vi "libssh2_session_last_errno.vi"(8 "error in (no error)":errorcluster, 11 "session":T1) -> (0 "error out":errorcluster, 2 "error code":i32)   [LabVIEW 2013, in "libssh2.lvlib"]
doc: "Get the last error code for a session."
uses:
  libssh2.lvlib
  Session Refnum.ctl
  Global Settings.vi
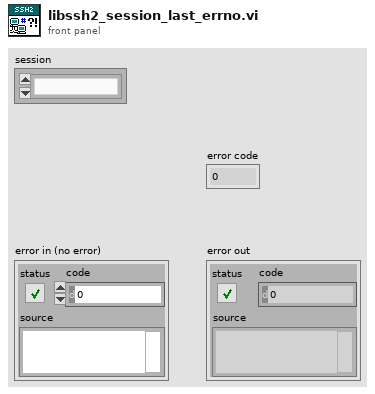
[diagram p1: front panel]
types:
  T1 = typedef "libssh2.lvlib/Session Refnum.ctl" = refnum<k1>
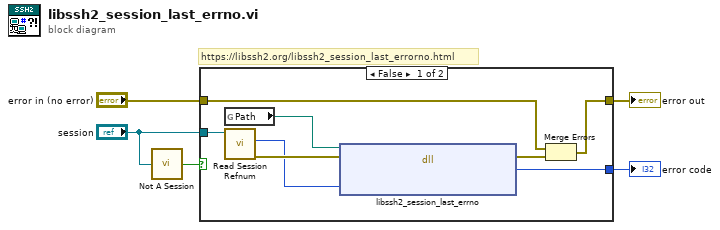
[diagram p0: block diagram]
diagram:
  # "https://libssh2.org/libssh2_session_last_errorno.html"
  n1 = call "Not A Session.vi"("session"="session") -> ("Not a Session?"=w1:bool)
  n2 = case shown="False" w1 {
    tunnel: [w8 w14] -> w5
    tunnel: [w13 _] -> w4
    tunnel: "error in (no error)" -> [w9 w14]
    tunnel: "session" -> [w11 _]
    frame False {
      n3 = global read "Global Settings.vi" "Path"() -> (w6:path)
      n4 = call "Read Session Refnum.vi"("session"=w11) -> ("error out"=w12:errorcluster, "LIBSSH2_SESSION*"=w10:u64)  [unwired: 6 in, 3 out]
      n5 = dll-call lib="?" fn="libssh2_session_last_errno"(path in=w6, error in=w12, "session"=w10) -> (error out=w7:errorcluster, "return value"=w13:i32)  [unwired: 2 in, 1 out]
      n6 = Merge Errors(w9, w7) -> (w8:errorcluster)
    }
    frame True {
    }
  }
  "error out" <- w5
  "error code" <- w4
